vi "AlazarTriggered.vi"(0 "Handle":u64, 1 "error in (no error)":errorcluster) -> (2 "Handle":u64, 3 "Triggered":bool, 5 "error out":errorcluster)   [LabVIEW 2018]
doc: "Determine if a board has triggered during the current acquisition."
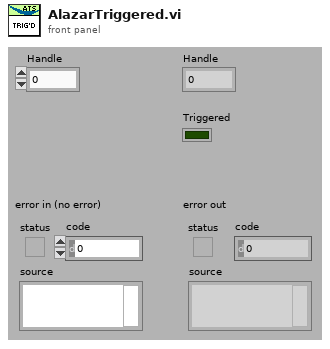
[diagram p1: front panel]
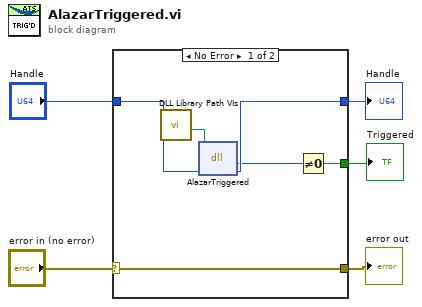
[diagram p0: block diagram]
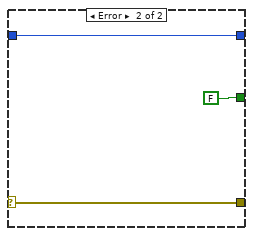
[diagram p2: hidden frame]
diagram:
  n1 = case shown="No Error" "error in (no error)" {
    selector: "error in (no error)" -> [w9 w14]
    tunnel: [w9 w14] -> w4
    tunnel: "Handle" -> [w11 w13]
    tunnel: [w10 w13] -> w2
    tunnel: [w7 FALSE] -> w1
    frame No Error {
      n2 = call "DLL Library Path VIs.vi"() -> ("Alazar"=w6:path)  [unwired: 9 in, 2 out]
      n3 = dll-call lib="C:/Project/SerialSectOCT - FFT GPU/SerialSectOCT/Labview Software/DLL/ATSApi.dll" fn="AlazarTriggered"(path in=w6, "handle"=w11) -> ("return type"=w8:u32, "handle"=w10:u64)  [unwired: 2 in, 2 out]
      n4 = Not Equal To 0?(x=w8) -> (x != 0?=w7:bool)
    }
    frame Error {
    }
  }
  "Handle" <- w2
  "error out" <- w4
  "Triggered" <- w1
